vi "String Word Wrapping with Get Nth Line Method.vi"() -> ()   [LabVIEW 2023]
doc: "The Get Nth Line method on the String class takes a line number as input and returns the text on that line. This provides a way to figure out where breaks in text should occur for word wrapping, a useful feature when trying to display text on one line at a time.\n\nThe example takes a piece of text from Input String and shows it in Output String. By loading the text into the Specific Width String first, the Get Nth Line method can be used to get a piece of text to match the Desired Width setting. Set the Desired Width before running this example. It will resize Specific Width String, which in turn will determine the amount of text shown in Output String. This method works even if Specific Width String is a hidden control."
panel:
  in  "Desired Width":u32(slide)=300 min=100 max=400 step=1 scale=100.0..400.0
  out "Output String":string
  out "Specific Width String":string
  in  "Input String":string="This text is from the LabVIEW Help topic on the Get Nth Line method. The Get Nth Line method gets the characters that make up the Nth line in a string control and returns the offsets in the original string in bytes.\n\nYou can use this method to determine how the text in a string control is word-wrapped. The position indexes are byte indexes. These are usually equivalent to character indexes, except when using text that has characters that use multiple bytes, such as Asian character sets."
  # "Overview: Demonstrates how the Get Nth Line method on the String class can be used to obtain the text displayed in a string control, one line at a time.\nInstructions:\n1. Specify a sufficiently lengthy Input String.\n2. Specify the Desired Width of the output string.\n3. Run the VI. The Specific Width String will be resized and populated with the value from the Input String. Then, each line from the Specific Width String will be displayed, one at a time, in the Output String indicator."
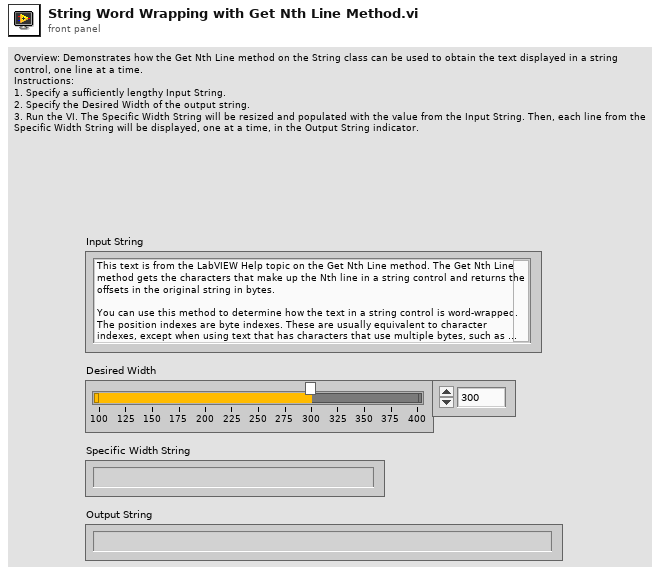
[diagram p1: front panel]
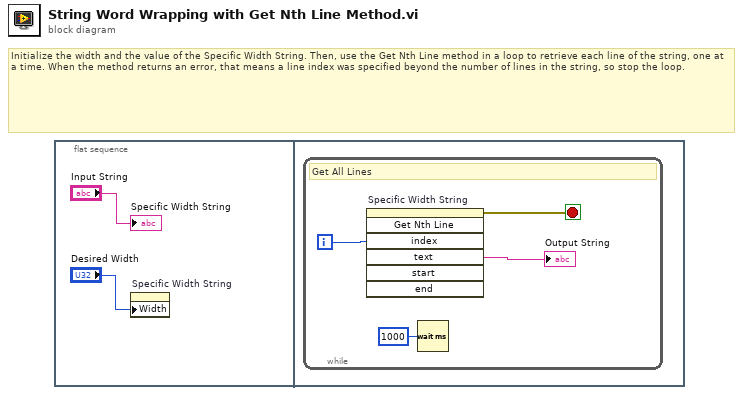
[diagram p0: block diagram]
diagram:
  # "Initialize the width and the value of the Specific Width String. Then, use the Get Nth Line method in a loop to retrieve each line of the string, one at a time. When the method returns an error, that means a line index was specified beyond the number of lines in the string, so stop the loop."
  n1 = flat-sequence {
    frame #0 {
      n2 = property on="Specific Width String" class="Str"("Width"="Desired Width") -> ()  [unwired: 2 in, 2 out]
      "Specific Width String" <- "Input String"
    }
    frame #1 {
      n3 = while {
        i -> [w6]
        stop <- w5 stop-if-true
        # "Get All Lines"
        n4 = invoke on="Specific Width String" class="String" method="Get Nth Line"("index"=w6) -> (error out=w5:errorcluster, "text"=→"Output String":string)  [unwired: 6 in, 5 out]
        n5 = Wait (ms)(milliseconds to wait=u32 1000) -> ()  [unwired: 1 out]
      }
    }
  }
